vi "Configure Waveform (Exponential).vi"(0 "VISA resource name":refnum<visa-resource-name>, 1 "Exponential Start Time (0.0 s)":dbl format="%^.3e", 2 "Exponential Start Level (0.0)":dbl format="%^.3e", 5 "Channel Name (1)":string="1", 7 "Exponential Time Constant (1.0)":dbl=1.0 format="%^.3e", 9 "Waveform Type (1: Voltage)":i32(ring)=1 items=["Voltage"=1, "Current"=0], 11 "error in (no error)":errorcluster {"code" format="%.0x"}, 12 "Exponential Total Time (1.0 s)":dbl=1.0 format="%^.3e", 13 "Exponential End Level (0.0)":dbl format="%^.3e") -> (4 "VISA resource name out":refnum<visa-resource-name>, 15 "error out":errorcluster {"code" format="%.0x"})   [LabVIEW 2018, in "Agilent N6700 Series.lvlib"]
doc: "Configures the exponential waveform.\n\n<b>Note:</b>\nThis VI only applies to the N6705B and N6705C DC Power Analyzer."
uses:
  Agilent N6700 Series.lvlib
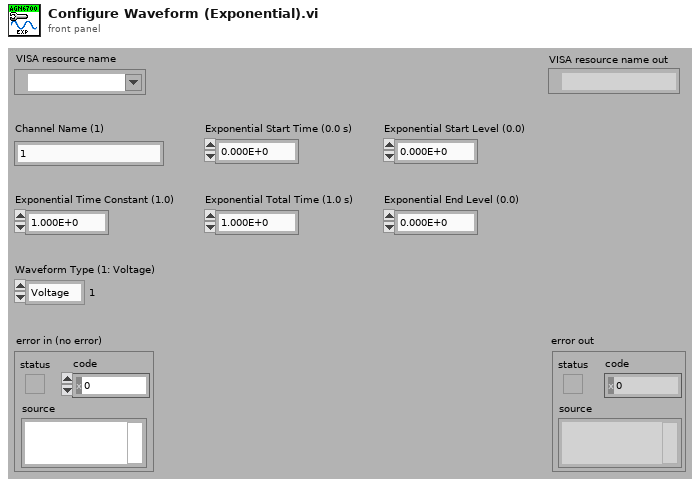
[diagram p1: front panel]
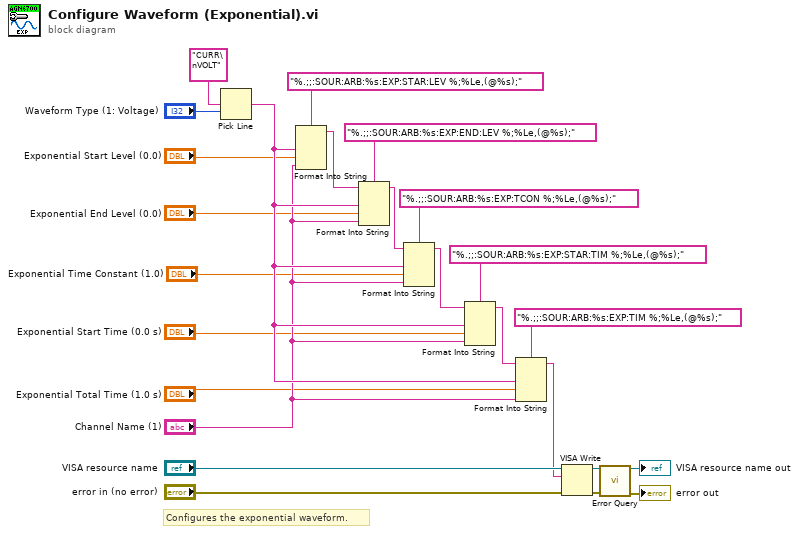
[diagram p0: block diagram]
diagram:
  # "Configures the exponential waveform."
  n1 = Pick Line(multi-line string="CURR\nVOLT", line index="Waveform Type (1: Voltage)") -> (output string=w14:string)  [unwired: 1 in]
  n2 = Format Into String(format string="%.;;:SOUR:ARB:%s:EXP:STAR:LEV %;%Le,(@%s);", w14, "Exponential Start Level (0.0)", "Channel Name (1)") -> (resulting string=w18:string)  [unwired: 2 in, 1 out]
  n3 = Format Into String(format string="%.;;:SOUR:ARB:%s:EXP:END:LEV %;%Le,(@%s);", initial string=w18, w14, "Exponential End Level (0.0)", "Channel Name (1)") -> (resulting string=w17:string)  [unwired: 1 in, 1 out]
  n4 = Format Into String(format string="%.;;:SOUR:ARB:%s:EXP:TCON %;%Le,(@%s);", initial string=w17, w14, "Exponential Time Constant (1.0)", "Channel Name (1)") -> (resulting string=w16:string)  [unwired: 1 in, 1 out]
  n5 = Format Into String(format string="%.;;:SOUR:ARB:%s:EXP:STAR:TIM %;%Le,(@%s);", initial string=w16, w14, "Exponential Start Time (0.0 s)", "Channel Name (1)") -> (resulting string=w15:string)  [unwired: 1 in, 1 out]
  n6 = Format Into String(format string="%.;;:SOUR:ARB:%s:EXP:TIM %;%Le,(@%s);", initial string=w15, w14, "Exponential Total Time (1.0 s)", "Channel Name (1)") -> (resulting string=w12:string)  [unwired: 1 in, 1 out]
  n7 = VISA Write(VISA resource name="VISA resource name", write buffer=w12, error in (no error)="error in (no error)") -> (VISA resource name out=w22:refnum<visa-resource-name>, error out=w21:errorcluster)  [unwired: 1 out]
  n8 = call "Error Query.vi"("VISA resource name"=w22, "error in (no error)"=w21) -> ("VISA resource name out"=→"VISA resource name out":refnum<visa-resource-name>, "error out"=→"error out":errorcluster)  [unwired: 10 in, 2 out]
